vi "front-back(SubVI).vi"(10 "distance":dbl, 11 "speed":dbl) -> ()   [LabVIEW 2016]
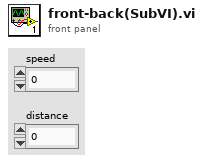
[diagram p1: front panel]
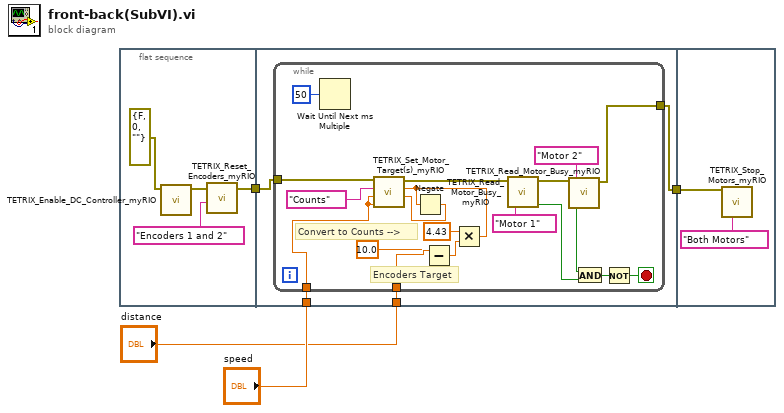
[diagram p0: block diagram]
diagram:
  n1 = flat-sequence {
    tunnel: [w7] -> w4
    tunnel: w4 -> [w12]
    tunnel: [w11] -> w3
    tunnel: "distance" -> [w10]
    tunnel: "speed" -> [w9]
    tunnel: w3 -> [w33]
    frame #0 {
      n2 = call <vilib>:"TETRIX_Enable_DC_Controller_myRIO.vi"("Error/Flow In"=errorcluster {"status"=FALSE, "code"=0, "source"=""}) -> ("Error/Flow Out"=w8:errorcluster)  [unwired: 6 in]
      n3 = call <vilib>:"TETRIX_Reset_Encoders_myRIO.vi"("Select Encoder"="Encoders 1 and 2", "Error/Flow In"=w8) -> ("Error/Flow Out"=w7:errorcluster)  [unwired: 5 in]
    }
    frame #1 {
      n4 = while {
        tunnel: w12 -> [w27]
        tunnel: [w18] -> w11
        tunnel: w10 -> [w15]
        tunnel: w9 -> [w17]
        stop <- w21 stop-if-true
        # "Convert to Counts -->"
        # "Encoders Target"
        n5 = Wait Until Next ms Multiple(millisecond multiple=u32 50) -> ()  [unwired: 1 out]
        n6 = Subtract(x=w15, y=10.0) -> (x-y=w13:dbl)
        n7 = Multiply(x=4.43, y=w13) -> (x*y=w19:dbl)
        n8 = Negate(x=w19) -> (-x=w26:dbl)
        n9 = call <vilib>:"TETRIX_Set_Motor_Target(s)_myRIO.vi"("Motor 2 Encoder Target"=w26, "Motor 1 Encoder Target"=w19, "Motor 2 Constant Speed (Degrees per Second)"=w17, "Motor 1 Contant Speed (Degrees per Second)"=w17, "Encoder Units"="Counts", "Error/Flow In"=w27) -> ("Error/Flow Out"=w29:errorcluster)  [unwired: 3 in]
        n10 = call <vilib>:"TETRIX_Read_Motor_Busy_myRIO.vi"("Select Channel"="Motor 1", "Error/Flow In"=w29) -> ("Error/Flow Out"=w25:errorcluster, "Motor Busy?"=w23:bool)  [unwired: 4 in]
        n11 = call <vilib>:"TETRIX_Read_Motor_Busy_myRIO.vi"("Select Channel"="Motor 2", "Error/Flow In"=w25) -> ("Error/Flow Out"=w18:errorcluster, "Motor Busy?"=w20:bool)  [unwired: 4 in]
        n12 = And(x=w20, y=w23) -> (x .and. y?=w22:bool)
        n13 = Not(x=w22) -> (.not. x?=w21:bool)
      }
    }
    frame #2 {
      n14 = call <vilib>:"TETRIX_Stop_Motors_myRIO.vi"("Select Channel"="Both Motors", "Error/Flow In"=w33) -> ()  [unwired: 5 in, 1 out]
    }
  }
